vi "Build WAV command substring.vi"(0 "System no.":i32=1 min=1 max=4 step=1, 2 "Waveform":u16(ring) items=["SIN", "POL", "TAN", "PNT", "SIN_P", "LIN", "RAMP", "NOISE", "SWEEP"], 3 "Axes to set":string[](array[string]), 4 "Append? (&)":bool, 5 "Add? (+)":bool, 6 "No. of digits":i16=3, 7 "error in (no error)":errorcluster, 8 "Xo":i32, 9 "N":i32=1000, 11 "Segment length":i32, 12 "PNT Parameters":cluster{"Ao..An-1":dbl[]}={"Ao..An-1"=[0.001, 0.002, 0.003, 0.004, 0.005, 0.006, 0.007, 0.008, 0.009, 0.01]} {"Ao..An-1" format="%.6f"}, 13 "SIN Parameters":T3={"A"=5.0, "N"=7692.0, "xo"=0.0, "Phi"=0.0, "B"=5.0} {"B" format="%.6f"; "Phi" format="%.6f"; "xo" format="%.6f"; "N" format="%.6f"; "A" format="%.6f"}, 14 "TAN Parameters":T3={"A"=10.0, "N"=6283.0, "xo"=0.0, "Phi"=0.0, "B"=0.0} {"B" format="%.6f"; "Phi" format="%.6f"; "xo" format="%.6f"; "N" format="%.6f"; "A" format="%.6f"}, 15 "POL Parameters":T2={"xo"=0.0, "Ao"=0.0, "A1"=0.01, "A2"=0.0, "A3"=0.0, "A4"=0.0, "A5"=0.0} {"A5" format="%.12f"; "A4" format="%.12f"; "A3" format="%.12f"; "A2" format="%.12f"; "A1" format="%.12f"; "Ao" format="%.12f"; "xo" format="%.12f"}, 16 "RAMP Parameters":cluster{"C":dbl, "J":dbl, "A":dbl, "O":dbl}={"C"=5.0, "J"=7692.0, "A"=0.0, "O"=0.0} {"O" format="%.6f"; "A" format="%.6f"; "J" format="%.6f"; "C" format="%.6f"}, 17 "SIN_P Parameters":cluster{"C":dbl, "A":dbl, "O":dbl}={"C"=5.0, "A"=7692.0, "O"=0.0} {"O" format="%.6f"; "A" format="%.6f"; "C" format="%.6f"}, 18 "LIN Parameters":cluster{"J":dbl, "A":dbl, "O":dbl}={"J"=5.0, "A"=7692.0, "O"=0.0} {"O" format="%.6f"; "A" format="%.6f"; "J" format="%.6f"}, 19 "NOISE Parameters":cluster{"A":dbl, "O":dbl}={"A"=5.0, "O"=0.0} {"O" format="%.6f"; "A" format="%.6f"}, 26 "SWEEP Parameters":T1={"Start"=0, "Stop"=0, "T"=0, "A"=5.0, "O"=0.0} {"O" format="%.6f"; "A" format="%.6f"}) -> (20 "WAV command substring":string, 27 "error out":errorcluster)   [LabVIEW 2026]
doc: "This VI builds a command substring for the WAV command. No. of digits is the number of digits after the decimal point in the parameter value(s) that will be sent. Sub-VI for WAV.vi."
uses:
  GeneralCommands/Controller names.ctl
  Communication/Syntax.ctl
  Communication/Global1.vi
  GeneralCommands/Global2 (Array).vi
panel:
  # "This vi builds a command substring for the WAV command."
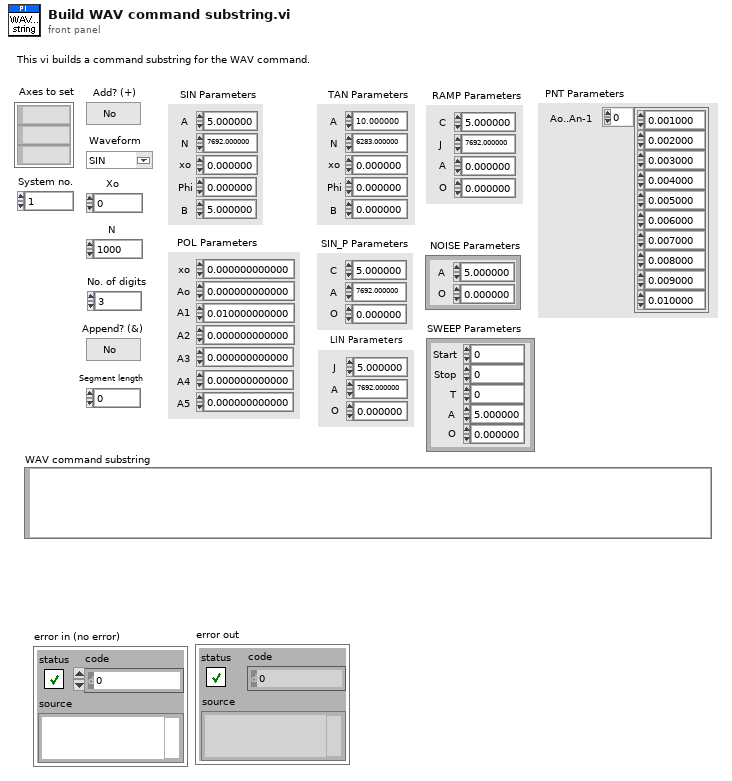
[diagram p1: front panel]
types:
  T1 = cluster{"Start":i32, "Stop":i32, "T":i32, "A":dbl, "O":dbl}
  T2 = cluster{"xo":dbl, "Ao":dbl, "A1":dbl, "A2":dbl, "A3":dbl, "A4":dbl, "A5":dbl}
  T3 = cluster{"A":dbl, "N":dbl, "xo":dbl, "Phi":dbl, "B":dbl}
  T4 = typedef "Syntax.ctl" = enum16{"GCS 1.0", "GCS 2.0", "GCS 3.0"}
  T5 = typedef "Controller names.ctl" = enum16{"None", "Analog", "C-702", "C-413", "C-414", "C-843", "C-843.PM", "C-844", "C-848", "C-865", "C-866", "C-867", "C-877", "C-880", "C-884", "C-885", "C-886", "C-887", "C-891", "E-135", "E-516", "E-517", "E-518", "E-709", "E-710", "E-712", "E-725", "E-727", "E-753", "E-754", "E-755", "E-761", "E-816", "E-861", "E-870", "E-871", "E-872", "E-873", "E-874", "F-206", "HydraPollux", "M-840", "M-850", "M-8X0", "Mercury", "Mercury_GCS", "PI_GCS2"}
  T6 = cluster{"Conn. axes":string[], "Controller name":T5}[]
  T7 = cluster{"Conn. axes":string[], "Controller name":T5}
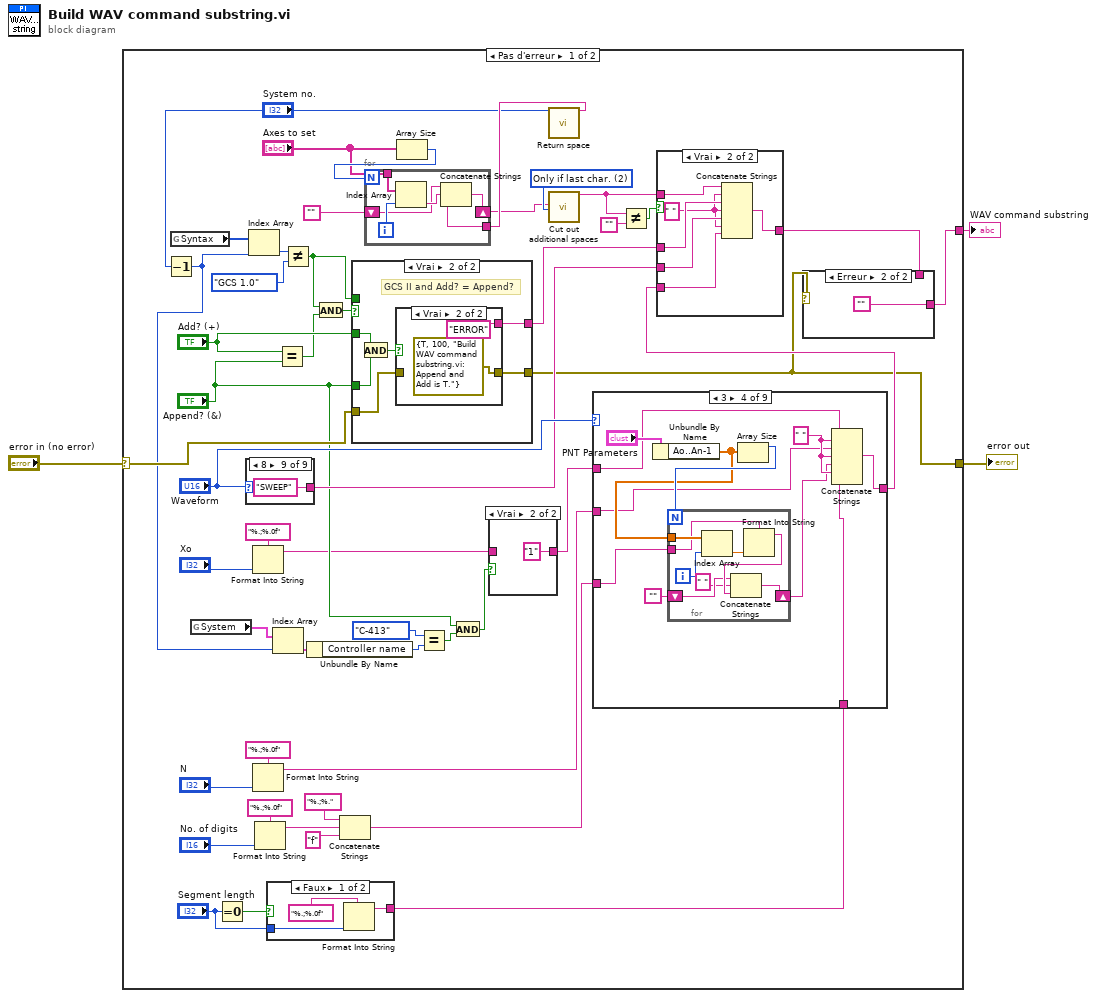
[diagram p0: block diagram]
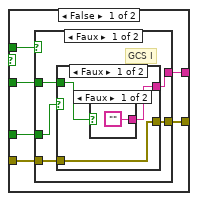
[diagram p4: hidden frame]
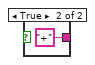
[diagram p5: hidden frame]
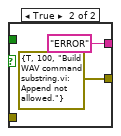
[diagram p6: hidden frame]
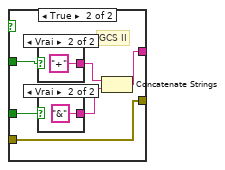
[diagram p7: hidden frame]
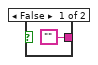
[diagram p8: hidden frame]
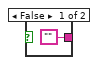
[diagram p9: hidden frame]
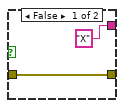
[diagram p10: hidden frame]
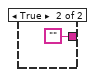
[diagram p11: hidden frame]
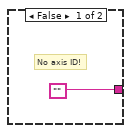
[diagram p12: hidden frame]
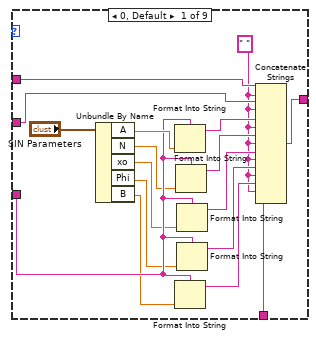
[diagram p13: hidden frame]
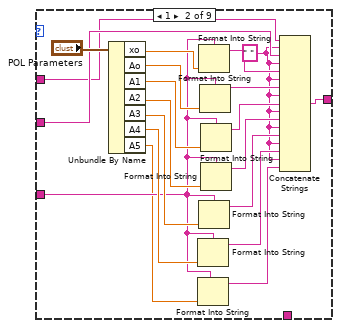
[diagram p14: hidden frame]
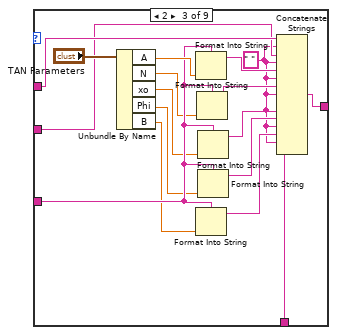
[diagram p15: hidden frame]
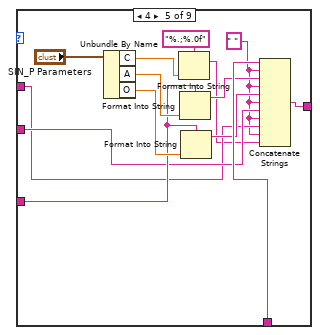
[diagram p16: hidden frame]
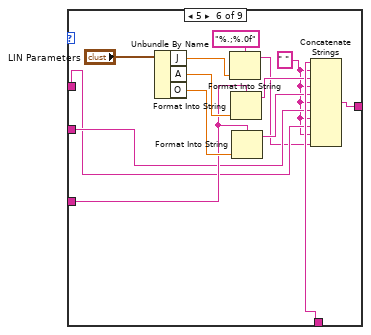
[diagram p17: hidden frame]
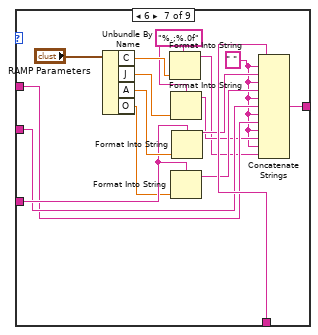
[diagram p18: hidden frame]
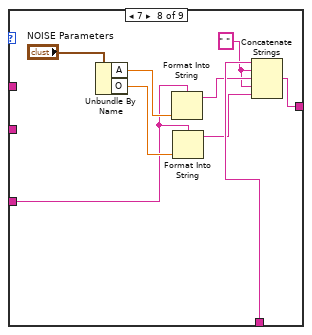
[diagram p19: hidden frame]
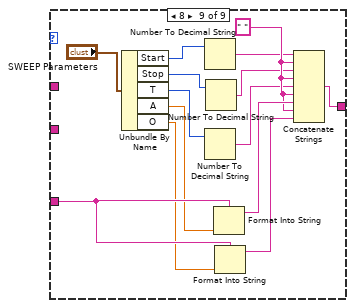
[diagram p20: hidden frame]
diagram:
  n1 = case shown="Pas d'erreur" "error in (no error)" {
    selector: "error in (no error)" -> [w19 w262]
    tunnel: [w18 w262] -> w2
    tunnel: [w17 ""] -> w1
    frame No Error {
      w30 = u16 2 items=["All Spaces", "Only if 1st char.", "Only if last char.", "Only if near \"=\"", "Only if 1st or last char.", "Only multiple"] ("Mode")
      n2 = Decrement(x="System no.") -> (x-1=w13:i32)
      n3 = global read "Global1.vi" "Syntax"() -> (w25:T4[])
      n4 = global read "Global2 (Array).vi" "System"() -> (w14:T6)
      n5 = Equal To 0?(x="Segment length") -> (x = 0?=w40:bool)
      n6 = case shown="8" "Waveform" {
        tunnel: ["SIN" "POL" "TAN" "PNT" "SIN_P" "LIN" "RAMP" "NOISE" "SWEEP"] -> w42
        frame 0, Default {
        }
        frame 1 {
        }
        frame 2 {
        }
        frame 3 {
        }
        frame 4 {
        }
        frame 5 {
        }
        frame 6 {
        }
        frame 7 {
        }
        frame 8 {
        }
      }
      n7 = Index Array(array=w25, index=w13) -> (element=w26:T4)
      n8 = Format Into String(format string="%.;%.0f" ("Format String"), "Xo") -> (resulting string=w6:string)  [unwired: 2 in, 1 out]
      n9 = Format Into String(format string="%.;%.0f" ("Format String"), "N") -> (resulting string=w33:string)  [unwired: 2 in, 1 out]
      n10 = Format Into String(format string="%.;%.0f" ("Format String"), "No. of digits") -> (resulting string=w36:string)  [unwired: 2 in, 1 out]
      n11 = case shown="Faux" w40 {
        tunnel: "Segment length" -> [w96 _]
        tunnel: [w95 ""] -> w32
        frame False {
          n12 = Format Into String(format string="%.;%.0f" ("Format String"), w96) -> (resulting string=w95:string)  [unwired: 2 in, 1 out]
        }
        frame True {
        }
      }
      n13 = Index Array(array=w14, index=w13) -> (element=w12:T7)
      n14 = Equal?(x="Add? (+)", y="Append? (&)") -> (x = y?=w20:bool)
      n15 = Not Equal?(x=w26, y=Syntax."GCS 1.0") -> (x != y?=w15:bool)
      n16 = Unbundle By Name(w12) -> ("Controller name"=w10:T5)
      n17 = And(x=w15, y=w20) -> (x .and. y?=w23:bool)
      n18 = Concatenate Strings("%.;%." ("Format String"), w36, "f" ("Format String")) -> (w34:string)
      n19 = case shown="Vrai" w23 {
        tunnel: [w60 w90] -> w22
        tunnel: "Add? (+)" -> [w62 w88]
        tunnel: "Append? (&)" -> [w61 w87]
        tunnel: w19 -> [w58 w86]
        tunnel: [w57 w85] -> w18
        tunnel: w15 -> [w59 _]
        frame False {
          n20 = case shown="Faux" w59 {
            tunnel: w62 -> [w63 w80]
            tunnel: w61 -> [w67 w79]
            tunnel: [w64 w76] -> w60
            tunnel: w58 -> [w66 w75]
            tunnel: [w65 w75] -> w57
            frame False {
              # "GCS I"
              n21 = case shown="Faux" w67 {
                tunnel: w66 -> [w68 _]
                tunnel: [w68 errorcluster {"status"=TRUE, "code"=100, "source"="Build WAV command substring.vi: Append not allowed."} ("error out")] -> w65
                tunnel: [w69 "ERROR"] -> w64
                tunnel: w63 -> [w70 _]
                frame False {
                  n22 = case shown="Faux" w70 {
                    tunnel: ["" "+"] -> w69
                    frame False {
                    }
                    frame True {
                    }
                  }
                }
                frame True {
                }
              }
            }
            frame True {
              # "GCS II"
              n23 = case shown="Vrai" w80 {
                tunnel: ["" "+"] -> w78
                frame False {
                }
                frame True {
                }
              }
              n24 = case shown="Vrai" w79 {
                tunnel: ["" "&"] -> w77
                frame False {
                }
                frame True {
                }
              }
              n25 = Concatenate Strings(w78, w77) -> (w76:string)
            }
          }
        }
        frame True {
          # "GCS II and Add? = Append?"
          n26 = And(x=w88, y=w87) -> (x .and. y?=w89:bool)
          n27 = case shown="Vrai" w89 {
            tunnel: ["X" "ERROR"] -> w90
            tunnel: w86 -> [w91 _]
            tunnel: [w91 errorcluster {"status"=TRUE, "code"=100, "source"="Build WAV command substring.vi: Append and Add is TRUE."} ("error out")] -> w85
            frame False {
            }
            frame True {
            }
          }
        }
      }
      n28 = Array Size(array="Axes to set") -> (size(s)=w52:i32)
      n29 = Equal?(x=Controller_names."C-413" ("System No. X"), y=w10) -> (x = y?=w9:bool)
      n30 = And(x="Append? (&)", y=w9) -> (x .and. y?=w7:bool)
      n31 = case shown="Vrai" w7 {
        tunnel: w6 -> [w53 _]
        tunnel: [w53 "1"] -> w5
        frame False {
        }
        frame True {
        }
      }
      n32 = call "Return space.vi"("System no."="System no.") -> ("String out"=w29:string)  [unwired: 1 in, 17 out]
      n33 = for {
        N: w52 -> [_]
        tunnel: "Axes to set" -> [w259]
        shift-right: [w258] -> w28
        shift-left: "" -> [w256]
        tunnel: w29 -> [w255]
        i -> [w260]
        n34 = Index Array(array=w259, index=w260) -> (element=w257:string)
        n35 = Concatenate Strings(w256, w257, w255) -> (w258:string)
      }
      n36 = call "Cut out additional spaces.vi"("String"=w28, "Mode"=w30) -> ("String out"=w27:string)  [unwired: 17 out]
      n37 = case shown="3" "Waveform" {
        tunnel: w34 -> [w120 w128 w158 w167 w187 w202 w217 w228 w244]
        tunnel: [w110 w132 w148 w162 w189 w203 w219 w229 w245] -> w31
        tunnel: w5 -> [w109 w124 w146 w165 w182 w196 w211 _ _]
        tunnel: w33 -> [w108 w125 w145 w163 w183 w197 w212 _ _]
        tunnel: w32 -> [w106 _ w143 w160 w186 w200 w215 w227 _]
        frame 0, Default {
          w107 = " " ("Substring")
          n38 = Unbundle By Name("SIN Parameters") -> ("A"=w121:dbl, "N"=w119:dbl, "xo"=w118:dbl, "Phi"=w117:dbl, "B"=w116:dbl)
          n39 = Format Into String(format string=w120, w121) -> (resulting string=w115:string)  [unwired: 2 in, 1 out]
          n40 = Format Into String(format string=w120, w116) -> (resulting string=w111:string)  [unwired: 2 in, 1 out]
          n41 = Format Into String(format string=w120, w119) -> (resulting string=w114:string)  [unwired: 2 in, 1 out]
          n42 = Format Into String(format string=w120, w118) -> (resulting string=w113:string)  [unwired: 2 in, 1 out]
          n43 = Format Into String(format string=w120, w117) -> (resulting string=w112:string)  [unwired: 2 in, 1 out]
          n44 = Concatenate Strings(w109, w107, w108, w107, w115, w107, w114, w107, w113, w107, w112, w107, w111, w107, w106) -> (w110:string)
        }
        frame 1 {
          w123 = " " ("Substring")
          n45 = Unbundle By Name("POL Parameters") -> ("xo"=w142:dbl, "Ao"=w141:dbl, "A1"=w140:dbl, "A2"=w139:dbl, "A3"=w138:dbl, "A4"=w130:dbl, "A5"=w127:dbl)
          n46 = Format Into String(format string=w128, w130) -> (resulting string=w129:string)  [unwired: 2 in, 1 out]
          n47 = Format Into String(format string=w128, w127) -> (resulting string=w126:string)  [unwired: 2 in, 1 out]
          n48 = Format Into String(format string=w128, w142) -> (resulting string=w137:string)  [unwired: 2 in, 1 out]
          n49 = Format Into String(format string=w128, w138) -> (resulting string=w133:string)  [unwired: 2 in, 1 out]
          n50 = Format Into String(format string=w128, w141) -> (resulting string=w136:string)  [unwired: 2 in, 1 out]
          n51 = Format Into String(format string=w128, w140) -> (resulting string=w135:string)  [unwired: 2 in, 1 out]
          n52 = Format Into String(format string=w128, w139) -> (resulting string=w134:string)  [unwired: 2 in, 1 out]
          n53 = Concatenate Strings(w124, w123, w125, w123, w137, w123, w136, w123, w135, w123, w134, w123, w133, w123, w129, w123, w126) -> (w132:string)
        }
        frame 2 {
          w144 = " " ("Substring")
          n54 = Unbundle By Name("TAN Parameters") -> ("A"=w159:dbl, "N"=w157:dbl, "xo"=w156:dbl, "Phi"=w155:dbl, "B"=w154:dbl)
          n55 = Format Into String(format string=w158, w159) -> (resulting string=w153:string)  [unwired: 2 in, 1 out]
          n56 = Format Into String(format string=w158, w154) -> (resulting string=w149:string)  [unwired: 2 in, 1 out]
          n57 = Format Into String(format string=w158, w157) -> (resulting string=w152:string)  [unwired: 2 in, 1 out]
          n58 = Format Into String(format string=w158, w156) -> (resulting string=w151:string)  [unwired: 2 in, 1 out]
          n59 = Format Into String(format string=w158, w155) -> (resulting string=w150:string)  [unwired: 2 in, 1 out]
          n60 = Concatenate Strings(w146, w144, w145, w144, w153, w144, w152, w144, w151, w144, w150, w144, w149, w144, w143) -> (w148:string)
        }
        frame 3 {
          w164 = " " ("Substring")
          n61 = Unbundle By Name("PNT Parameters") -> ("Ao..An-1"=w168:dbl[])
          n62 = Array Size(array=w168) -> (size(s)=w169:i32)
          n63 = for {
            N: w169 -> [_]
            tunnel: w168 -> [w177]
            tunnel: w167 -> [w175]
            shift-right: [w174] -> w161
            shift-left: "" ("Substring") -> [w172]
            i -> [w178]
            n64 = Index Array(array=w177, index=w178) -> (element=w176:dbl)
            n65 = Format Into String(format string=w175, w176) -> (resulting string=w173:string)  [unwired: 2 in, 1 out]
            n66 = Concatenate Strings(w172, " " ("Substring"), w173) -> (w174:string)
          }
          n67 = Concatenate Strings(w165, w164, w163, w164, w161, w164, w160) -> (w162:string)
        }
        frame 4 {
          w181 = " " ("Substring")
          n68 = Unbundle By Name("SIN_P Parameters") -> ("C"=w192:dbl, "A"=w191:dbl, "O"=w190:dbl)
          n69 = Format Into String(format string="%.;%.0f", w192) -> (resulting string=w180:string)  [unwired: 2 in, 1 out]
          n70 = Format Into String(format string=w187, w191) -> (resulting string=w185:string)  [unwired: 2 in, 1 out]
          n71 = Format Into String(format string=w187, w190) -> (resulting string=w184:string)  [unwired: 2 in, 1 out]
          n72 = Concatenate Strings(w186, w181, w185, w181, w184, w181, w183, w181, w182, w181, w180) -> (w189:string)
        }
        frame 5 {
          w195 = " " ("Substring")
          n73 = Unbundle By Name("LIN Parameters") -> ("J"=w206:dbl, "A"=w205:dbl, "O"=w204:dbl)
          n74 = Format Into String(format string="%.;%.0f", w206) -> (resulting string=w194:string)  [unwired: 2 in, 1 out]
          n75 = Format Into String(format string=w202, w205) -> (resulting string=w199:string)  [unwired: 2 in, 1 out]
          n76 = Format Into String(format string=w202, w204) -> (resulting string=w198:string)  [unwired: 2 in, 1 out]
          n77 = Concatenate Strings(w200, w195, w199, w195, w198, w195, w197, w195, w196, w195, w194) -> (w203:string)
        }
        frame 6 {
          w207 = "%.;%.0f" ("format string")
          w209 = " " ("Substring")
          n78 = Unbundle By Name("RAMP Parameters") -> ("C"=w222:dbl, "J"=w221:dbl, "A"=w220:dbl, "O"=w216:dbl)
          n79 = Format Into String(format string=w207, w222) -> (resulting string=w208:string)  [unwired: 2 in, 1 out]
          n80 = Format Into String(format string=w207, w221) -> (resulting string=w210:string)  [unwired: 2 in, 1 out]
          n81 = Format Into String(format string=w217, w216) -> (resulting string=w213:string)  [unwired: 2 in, 1 out]
          n82 = Format Into String(format string=w217, w220) -> (resulting string=w214:string)  [unwired: 2 in, 1 out]
          n83 = Concatenate Strings(w215, w209, w214, w209, w213, w209, w212, w209, w211, w209, w210, w209, w208) -> (w219:string)
        }
        frame 7 {
          w224 = " " ("Substring")
          n84 = Unbundle By Name("NOISE Parameters") -> ("A"=w231:dbl, "O"=w230:dbl)
          n85 = Format Into String(format string=w228, w231) -> (resulting string=w226:string)  [unwired: 2 in, 1 out]
          n86 = Format Into String(format string=w228, w230) -> (resulting string=w225:string)  [unwired: 2 in, 1 out]
          n87 = Concatenate Strings(w227, w224, w226, w224, w225) -> (w229:string)
        }
        frame 8 {
          w238 = " " ("Substring")
          n88 = Unbundle By Name("SWEEP Parameters") -> ("Start"=w237:i32, "Stop"=w236:i32, "T"=w235:i32, "A"=w240:dbl, "O"=w239:dbl)
          n89 = Number To Decimal String(number=w237) -> (decimal integer string=w234:string)  [unwired: 1 out]
          n90 = Number To Decimal String(number=w235) -> (decimal integer string=w232:string)  [unwired: 1 out]
          n91 = Number To Decimal String(number=w236) -> (decimal integer string=w233:string)  [unwired: 1 out]
          n92 = Format Into String(format string=w244, w240) -> (resulting string=w243:string)  [unwired: 2 in, 1 out]
          n93 = Format Into String(format string=w244, w239) -> (resulting string=w242:string)  [unwired: 2 in, 1 out]
          n94 = Concatenate Strings(w234, w238, w233, w238, w232, w238, w243, w238, w242) -> (w245:string)
        }
      }
      n95 = Not Equal?(x=w27, y="") -> (x != y?=w43:bool)
      n96 = case shown="Vrai" w43 {
        tunnel: w27 -> [_ w101]
        tunnel: w42 -> [_ w105]
        tunnel: ["" w104] -> w16
        tunnel: w22 -> [_ w103]
        tunnel: w31 -> [_ w102]
        frame False {
          # "No axis ID!"
        }
        frame True {
          w100 = " "
          n97 = Concatenate Strings(w101, w100, w103, w100, w105, w100, w102) -> (w104:string)
        }
      }
      n98 = case shown="Erreur" w18 {
        tunnel: [w55 ""] -> w17
        tunnel: w16 -> [w55 _]
        frame No Error {
        }
        frame Error {
        }
      }
    }
    frame Error {
    }
  }
  "error out" <- w2
  "WAV command substring" <- w1
